vi "check_range.vi"(2 "max":i16, 3 "min":i16, 4 "x":i16) -> (1 "checked x":i16)   [LabVIEW 2016]
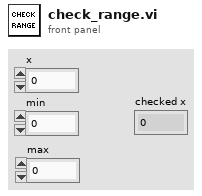
[diagram p1: front panel]
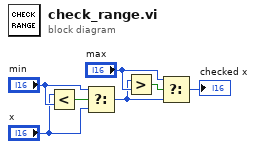
[diagram p0: block diagram]
diagram:
  n1 = Less?(x="x", y="min") -> (x < y?=w7:bool)
  n2 = Select(t="min", s=w7, f="x") -> (s? t:f=w1:i16)
  n3 = Greater?(x=w1, y="max") -> (0:w4:bool)
  n4 = Select(t="max", s=w4, f=w1) -> (s? t:f=→"checked x":i16)
